vi "Teleop.vi"(10 "Match Info":T1={"Autonomous Elapsed Seconds"=0.0, "TeleOp Elapsed Seconds"=0.0, "Disabled Elapsed Seconds"=0.0, "Visited Autonomous"=FALSE, "Visited TeleOp"=FALSE, "Visited Disabled"=FALSE, "Autonomous Settings"={"Autonomous Style"=enum."Independent", "VI Refnum"=refnum}}, 11 "Call Context":T2) -> ()   [LabVIEW 2017]
doc: "This VI is called for each TeleOp packet received from the DS where the robot is not disabled. It is often used to read from the joysticks and update I/O or to update setpoints for timed control loops. It should complete and return within 20 milliseconds or it may miss DS packets."
uses:
  <vilib>/Rock Robotics/WPI/DriverStation/WPI_DriverStationDerivedRobotMode.ctl
  <vilib>/Rock Robotics/WPI/DriverStation/WPI_DriverStationMatch Info.ctl
  <vilib>/Rock Robotics/WPI/Utilities/WPI_GetSetVariantRefNum.vi
  <vilib>/Rock Robotics/Network Tables/NT Write Boolean Array.vi
  <vilib>/Rock Robotics/Network Tables/NT Write Numeric Array.vi
  <vilib>/Rock Robotics/Network Tables/NT Write Boolean.vi
  <vilib>/Rock Robotics/Network Tables/NT Read Boolean.vi
  <vilib>/Rock Robotics/Network Tables/NT Read Number.vi
panel:
  out "Sample Slider 0":dbl(slide) scale=0.0..5.0
  out "Sample Boolean 1":bool
  out "Sample Boolean 0":bool
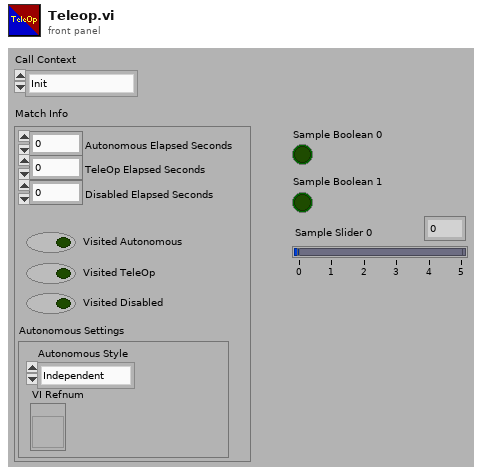
[diagram p1: front panel]
types:
  T1 = typedef "WPI_DriverStationMatch Info.ctl" = cluster{"Autonomous Elapsed Seconds":dbl, "TeleOp Elapsed Seconds":dbl, "Disabled Elapsed Seconds":dbl, "Visited Autonomous":bool, "Visited TeleOp":bool, "Visited Disabled":bool, "Autonomous Settings":cluster{"Autonomous Style":enum16{"Iterative", "Independent"}, "VI Refnum":refnum<vi>}}
  T2 = typedef "WPI_DriverStationDerivedRobotMode.ctl" = enum16{"Init", "Execute", "Stop"}
  T3 = typedef "WPI_RobotDriveDevRef.ctl" = cluster{"DevStatus":errorcluster, "Motors[]":T4[], "Square Inputs":bool, "Max Output":dbl}
  T4 = typedef "WPI_MotorControlDeviceRef.ctl" = cluster{"DeviceStatus":errorcluster, "Type":T5, "PWM":cluster{"PWM Channel":T6, "DeadBand":T7}, "CAN":cluster{"Device Number":u8, "SetOutput VI Ref":variant, "GetOutput VI Ref":variant, "Enable VI Ref":variant, "Disable VI Ref":variant, "Data":variant}, "Invert":bool, "DIO PWM":cluster{"PWM \"Enable\" Channel":T6, "DIOChannel":T8, "PWM Rate":dbl}}
  T5 = typedef "WPI_MotorControlType.ctl" = enum16{"PWM", "CAN", "DIO PWM"}
  T6 = typedef "FPGA_DIOPWMChannel.ctl" = enum8{"PWM 0", "PWM 1", "PWM 2", "PWM 3", "PWM 4", "PWM 5", "PWM 6", "PWM 7", "PWM 8", "PWM 9", "PWM MXP 0", "PWM MXP 1", "PWM MXP 2", "PWM MXP 3", "PWM MXP 4", "PWM MXP 5", "PWM MXP 6", "PWM MXP 7", "PWM MXP 8", "PWM MXP 9", "Invalid"}
  T7 = typedef "WPI_PWMDeadband.ctl" = cluster{"Name":string, "maxPositivePwm":i32, "minPositivePwm":i32, "centerPwm":i32, "maxNegativePwm":i32, "minNegativePwm":i32, "angularRange":u16}
  T8 = typedef "FPGA_DIOChannel.ctl" = enum8{"DIO 0", "DIO 1", "DIO 2", "DIO 3", "DIO 4", "DIO 5", "DIO 6", "DIO 7", "DIO 8", "DIO 9", "DIO MXP 0", "DIO MXP 1", "DIO MXP 2", "DIO MXP 3", "DIO MXP 4", "DIO MXP 5", "DIO MXP 6", "DIO MXP 7", "DIO MXP 8", "DIO MXP 9", "DIO MXP 10", "DIO MXP 11", "DIO MXP 12", "DIO MXP 13", "DIO MXP 14", "DIO MXP 15", "SPI Port CS1", "SPI Port CS2", "SPI Port CS3", "SPI Port MISO", "SPI Port MOSI", "Invalid"}
  T9 = typedef "WPI_JoystickDevRef.ctl" = cluster{"Device":T10}
  T10 = typedef "WPI_JoystickDeviceEnum.ctl" = enum16{"USB 0", "USB 1", "USB 2", "USB 3", "USB 4", "USB 5"}
  T11 = typedef "WPI_SwitchDevRef.ctl" = cluster{"DevStatus":errorcluster, "DIO Channel":T8, "CntIndex":T12, "Normally Closed":bool}
  T12 = typedef "FPGA_CounterCtrSystemIndex.ctl" = enum8{"Ctr 0", "Ctr 1", "Ctr 2", "Ctr 3", "Ctr 4", "Ctr 5", "Ctr 6", "Ctr 7", "Invalid"}
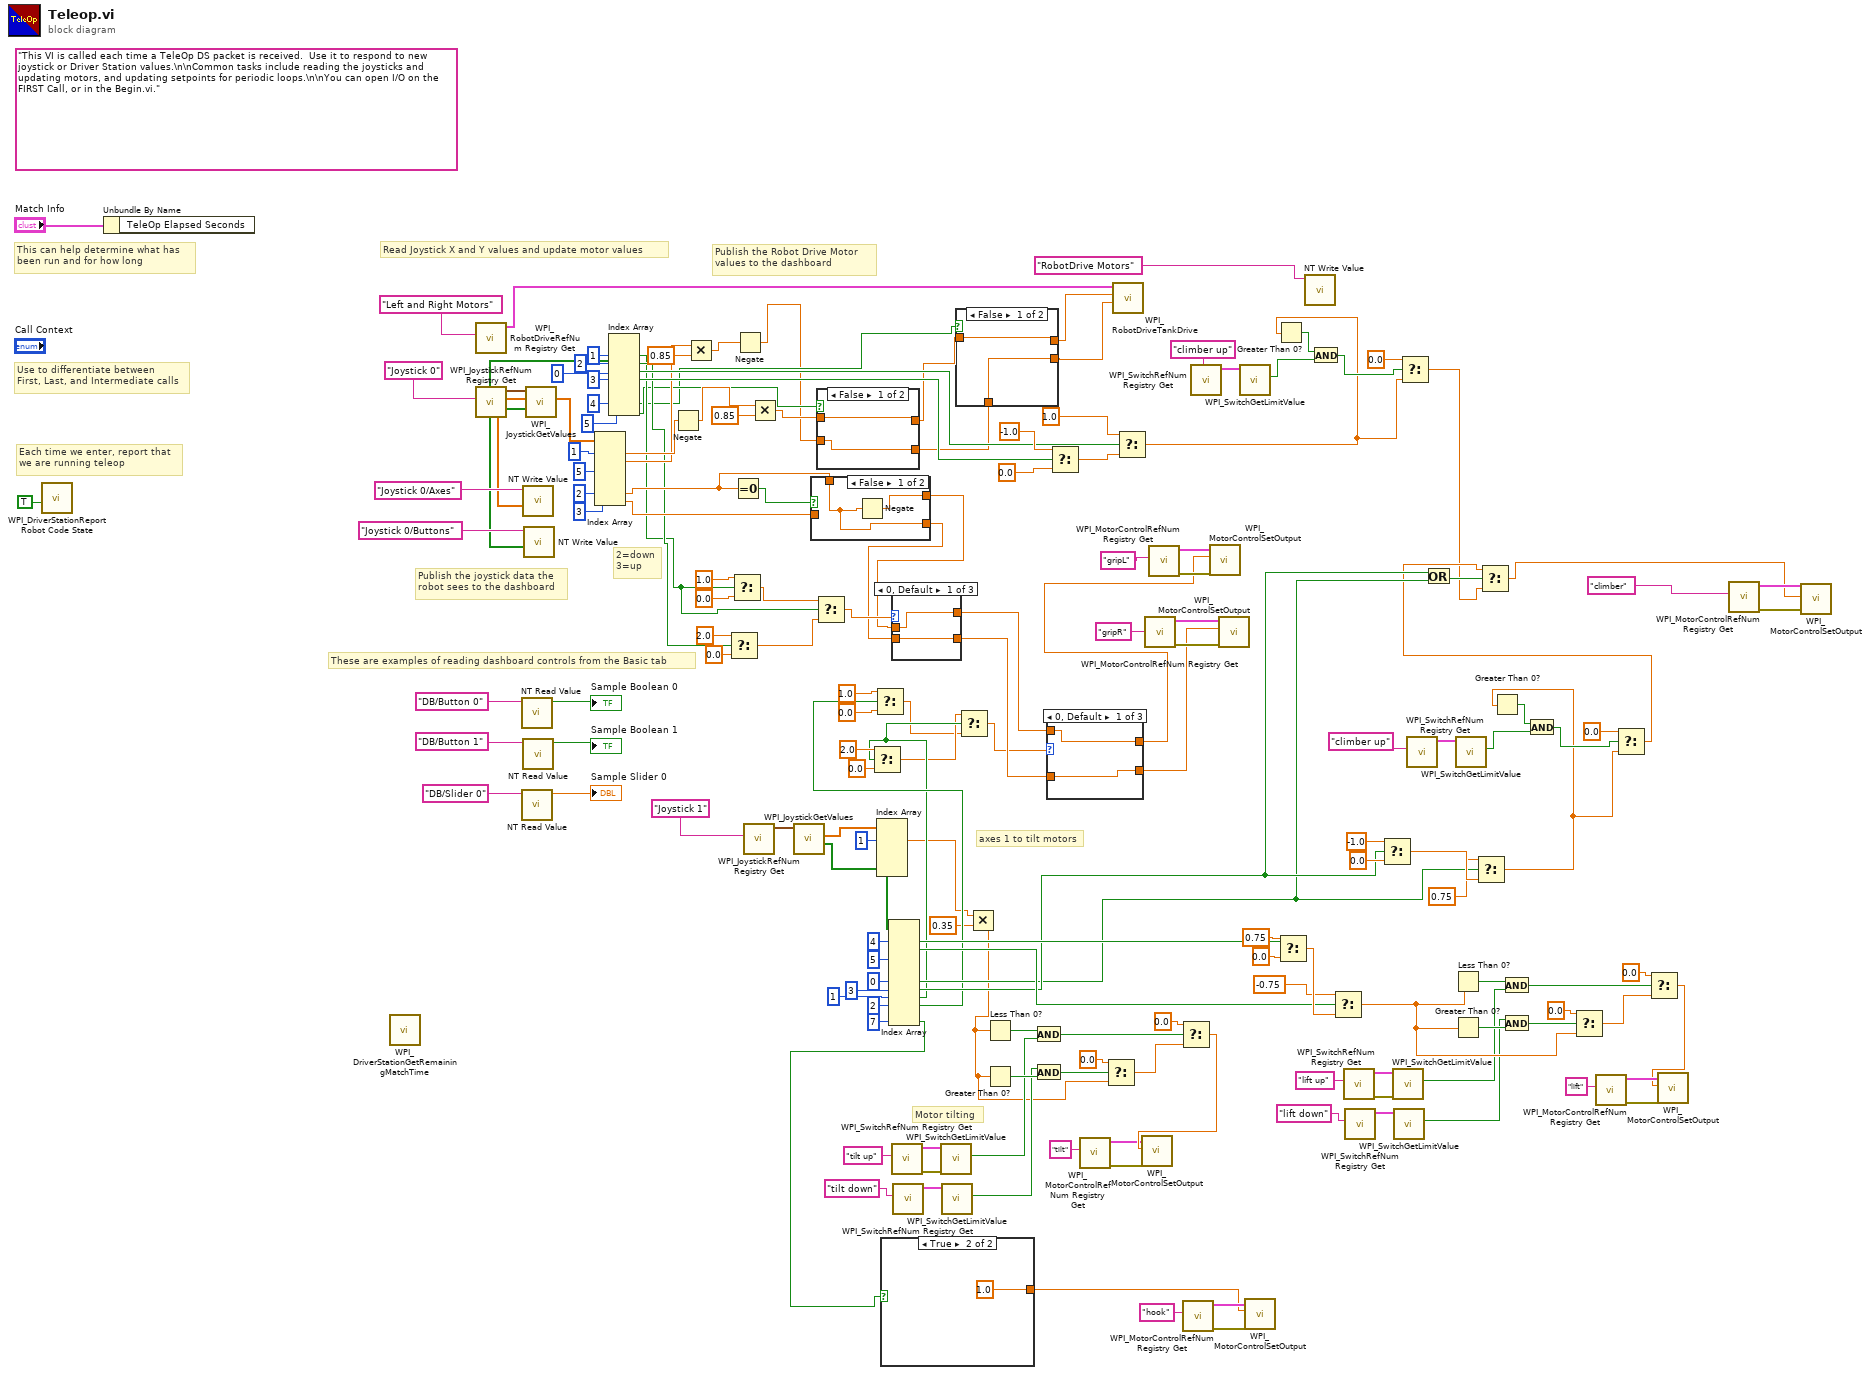
[diagram p0: block diagram]
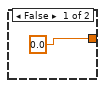
[diagram p2: hidden frame]
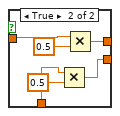
[diagram p3: hidden frame]
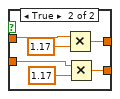
[diagram p4: hidden frame]
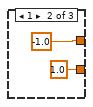
[diagram p5: hidden frame]
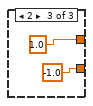
[diagram p6: hidden frame]
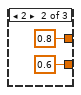
[diagram p7: hidden frame]
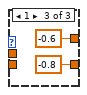
[diagram p8: hidden frame]
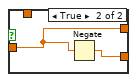
[diagram p9: hidden frame]
diagram:
  (unwired) "This VI is called each time a TeleOp DS packet is received.  Use it to respond to new joystick or Driver Station values.\n\nCommon tasks include reading the joysticks and updating motors, and updating setpoints for periodic loops.\n\nYou can open I/O on the FIRST Call, or in the Begin.vi."
  # "Motor tilting"
  # "axes 1 to tilt motors"
  # "2=down\n3=up"
  # "These are examples of reading dashboard controls from the Basic tab"
  # "Publish the Robot Drive Motor\nvalues to the dashboard"
  # "Publish the joystick data the\nrobot sees to the dashboard"
  # "Each time we enter, report that\nwe are running teleop"
  # "Use to differentiate between\nFirst, Last, and Intermediate calls"
  # "This can help determine what has\nbeen run and for how long"
  # "Read Joystick X and Y values and update motor values"
  n1 = call <vilib>:"WPI_DriverStationReport Robot Code State.vi"("TeleOp"=TRUE ("Autonomous")) -> ()  [unwired: 10 in, 1 out]
  n2 = Unbundle By Name("Match Info") -> ()  [unwired: 1 out]
  n3 = call <vilib>:"WPI_DriverStationGetRemainingMatchTime.vi"() -> ()  [unwired: 10 in, 2 out]
  n4 = call <vilib>:"WPI_RobotDriveRefNum Registry Get.vi"("refnum name"="Left and Right Motors") -> ("RobotDriveDevRef"=w1:T3)  [unwired: 1 in, 9 out]
  n5 = call <vilib>:"WPI_JoystickRefNum Registry Get.vi"("refnum name"="Joystick 0") -> ("JoystickDevRef"=w167:T9)  [unwired: 1 in, 9 out]
  n6 = call-poly <vilib>:"NT Read Value.vi"("Name"="DB/Button 0" ("refnum name")) -> ("Boolean"=→"Sample Boolean 0":bool)  [unwired: 9 in, 1 out]
  n7 = call-poly <vilib>:"NT Read Value.vi"("Name"="DB/Slider 0" ("refnum name")) -> ("Numeric"=→"Sample Slider 0":dbl)  [unwired: 9 in, 1 out]
  n8 = call-poly <vilib>:"NT Read Value.vi"("Name"="DB/Button 1" ("refnum name")) -> ("Boolean"=→"Sample Boolean 1":bool)  [unwired: 9 in, 1 out]
  n9 = call <vilib>:"WPI_JoystickGetValues.vi"("JoystickDevRef"=w167) -> ("Buttons"=w151:bool[], "Axes"=w163:dbl[])  [unwired: 6 in, 3 out]
  n10 = call-poly <vilib>:"NT Write Value.vi"("Numeric Array"=w163, "Name"="Joystick 0/Axes") -> ()  [unwired: 9 in, 1 out]
  n11 = call-poly <vilib>:"NT Write Value.vi"("Boolean Array"=w151, "Name"="Joystick 0/Buttons") -> ()  [unwired: 9 in, 1 out]
  n12 = Index Array(array=w163, index #1=1 ("index"), index #2=5 ("index"), index #6=2 ("index"), index #7=3 ("index")) -> (element #1=w138:dbl, element #2=w129:dbl, element #6=w132:dbl, element #7=w133:dbl)  [unwired: 3 in, 3 out]
  n13 = Index Array(array=w151, index #1=1 ("index"), index #2=2 ("index"), index #3=0 ("index"), index #4=3 ("index"), index #7=4 ("index"), index #8=5 ("index")) -> (element #1=w58:bool, element #2=w61:bool, element #3=w139:bool, element #4=w146:bool, element #7=w44:bool, element #8=w47:bool)  [unwired: 2 in, 2 out]
  n14 = Negate(x=w138) -> (-x=w131:dbl)
  n15 = Multiply(x=w129, y=0.85) -> (x*y=w127:dbl)
  n16 = Select(t=2.0, s=w61, f=0.0) -> (s? t:f=w62:dbl)
  n17 = Select(t=1.0, s=w58, f=0.0) -> (s? t:f=w63:dbl)
  n18 = Equal To 0?(x=w132) -> (x = 0?=w134:bool)
  n19 = Negate(x=w127) -> (-x=w43:dbl)
  n20 = call <vilib>:"WPI_JoystickRefNum Registry Get.vi"("refnum name"="Joystick 1") -> ("JoystickDevRef"=w154:T9)  [unwired: 1 in, 9 out]
  n21 = Multiply(x=w131, y=0.85) -> (x*y=w46:dbl)
  n22 = call <vilib>:"WPI_JoystickGetValues.vi"("JoystickDevRef"=w154) -> ("Buttons"=w97:bool[], "Axes"=w153:dbl[])  [unwired: 6 in, 3 out]
  n23 = case shown="False" w134 {
    tunnel: [w172 w174] -> w56
    tunnel: w133 -> [_ w174]
    tunnel: w132 -> [w171 _]
    tunnel: [w171 w173] -> w55
    frame False {
      n24 = Negate(x=w171) -> (-x=w172:dbl)
    }
    frame True {
      n25 = Negate(x=w174) -> (-x=w173:dbl)
    }
  }
  n26 = Select(t=w63, s=w58, f=w62) -> (s? t:f=w57:dbl)
  n27 = case shown="False" w47 {
    tunnel: w46 -> [w176 w182]
    tunnel: [w176 w180] -> w45
    tunnel: w43 -> [w175 w178]
    tunnel: [w175 w177] -> w2
    frame False {
    }
    frame True {
      n28 = Multiply(x=w182, y=1.17) -> (x*y=w180:dbl)
      n29 = Multiply(x=w178, y=1.17) -> (x*y=w177:dbl)
    }
  }
  n30 = Index Array(array=w153, index #1=1 ("index")) -> (element #1=w7:dbl)  [unwired: 4 in, 4 out]
  n31 = Index Array(array=w97, index #1=4 ("index"), index #2=5 ("index"), index #6=0 ("index"), index #7=3 ("index"), index #8=1 ("index"), index #9=2 ("index"), index #11=7 ("index")) -> (element #1=w94:bool, element #2=w93:bool, element #6=w74:bool, element #7=w75:bool, element #8=w36:bool, element #9=w37:bool, element #11=w9:bool)  [unwired: 4 in, 4 out]
  n32 = Select(t=2.0, s=w36, f=0.0) -> (s? t:f=w15:dbl)
  n33 = Select(t=1.0, s=w37, f=0.0) -> (s? t:f=w14:dbl)
  n34 = case shown="True" w9 {
    tunnel: [0.0 ("Output") 1.0 ("Output")] -> w8
    frame False {
    }
    frame True {
    }
  }
  n35 = case shown="0, Default" w57 {
    tunnel: [w186 0.8 ("upper limit") -0.6 ("upper limit")] -> w52
    tunnel: w56 -> [w186 _ _]
    tunnel: [w185 0.6 ("upper limit") -0.8 ("upper limit")] -> w50
    tunnel: w55 -> [w185 _ _]
    frame 0, Default {
    }
    frame 2 {
    }
    frame 1 {
    }
  }
  n36 = call <vilib>:"WPI_SwitchRefNum Registry Get.vi"("refnum name"="tilt up") -> ("error out"=w33:errorcluster, "SwitchDevRef"=w32:T11)  [unwired: 9 in]
  n37 = call <vilib>:"WPI_SwitchRefNum Registry Get.vi"("refnum name"="tilt down") -> ("SwitchDevRef"=w31:T11)  [unwired: 9 in, 1 out]
  n38 = call <vilib>:"WPI_SwitchGetLimitValue.vi"("error in (no error)"=w33, "SwitchDevRef"=w32) -> ("Switch Pressed"=w18:bool)  [unwired: 7 in, 2 out]
  n39 = call <vilib>:"WPI_SwitchGetLimitValue.vi"("SwitchDevRef"=w31) -> ("Switch Pressed"=w19:bool)  [unwired: 8 in, 2 out]
  n40 = case shown="False" w44 {
    tunnel: w45 -> [w192 w198]
    tunnel: [w192 w196] -> w4
    tunnel: [w191 w193] -> w3
    tunnel: w2 -> [w191 w194]
    frame False {
    }
    frame True {
      n41 = Multiply(x=w194, y=0.5) -> (x*y=w193:dbl)
      n42 = Multiply(x=w198, y=0.5) -> (x*y=w196:dbl)
    }
  }
  n43 = Select(t=w15, s=w36, f=w14) -> (s? t:f=w35:dbl)
  n44 = Multiply(x=w7, y=0.35) -> (x*y=w6:dbl)
  n45 = Less Than 0?(x=w6) -> (x < 0?=w23:bool)
  n46 = Greater Than 0?(x=w6) -> (x > 0?=w24:bool)
  n47 = And(x=w23, y=w18) -> (x .and. y?=w25:bool)
  n48 = And(x=w19, y=w24) -> (x .and. y?=w26:bool)
  n49 = case shown="0, Default" w35 {
    tunnel: [w199 -1.0 ("upper limit") 1.0 ("upper limit")] -> w53
    tunnel: w52 -> [w199 _ _]
    tunnel: [w200 1.0 ("upper limit") -1.0 ("upper limit")] -> w51
    tunnel: w50 -> [w200 _ _]
    frame 0, Default {
    }
    frame 1 {
    }
    frame 2 {
    }
  }
  n50 = Select(t=-1.0, s=w146, f=0.0) -> (s? t:f=w143:dbl)
  n51 = call <vilib>:"WPI_MotorControlRefNum Registry Get.vi"("refnum name"="tilt") -> ("error out"=w27:errorcluster, "MotorControlDevRef"=w16:T4)  [unwired: 9 in]
  n52 = Select(t=0.0, s=w26, f=w6) -> (s? t:f=w20:dbl)
  n53 = call <vilib>:"WPI_RobotDriveTankDrive.vi"("Right axis value"=w3, "Left axis value"=w4, "RobotDriveDevRef"=w1) -> ()  [unwired: 6 in, 3 out]
  n54 = Select(t=1.0, s=w139, f=w143) -> (s? t:f=w120:dbl)
  n55 = call <vilib>:"WPI_MotorControlRefNum Registry Get.vi"("refnum name"="gripR") -> ("error out"=w69:errorcluster, "MotorControlDevRef"=w49:T4)  [unwired: 9 in]
  n56 = call <vilib>:"WPI_MotorControlRefNum Registry Get.vi"("refnum name"="gripL") -> ("error out"=w135:errorcluster, "MotorControlDevRef"=w136:T4)  [unwired: 9 in]
  n57 = Select(t=0.0, s=w25, f=w20) -> (s? t:f=w17:dbl)
  n58 = call <vilib>:"WPI_MotorControlSetOutput.vi"("error in (no error)"=w27, "Output"=w17, "MotorControlDevRef"=w16) -> ()  [unwired: 6 in, 3 out]
  n59 = call <vilib>:"WPI_MotorControlRefNum Registry Get.vi"("refnum name"="hook") -> ("error out"=w12:errorcluster, "MotorControlDevRef"=w11:T4)  [unwired: 9 in]
  n60 = call <vilib>:"WPI_SwitchRefNum Registry Get.vi"("refnum name"="climber up") -> ("SwitchDevRef"=w126:T11)  [unwired: 9 in, 1 out]
  n61 = call <vilib>:"WPI_MotorControlSetOutput.vi"("error in (no error)"=w135, "Output"=w53, "MotorControlDevRef"=w136) -> ()  [unwired: 6 in, 3 out]
  n62 = call <vilib>:"WPI_MotorControlSetOutput.vi"("error in (no error)"=w69, "Output"=w51, "MotorControlDevRef"=w49) -> ()  [unwired: 6 in, 3 out]
  n63 = call <vilib>:"WPI_SwitchGetLimitValue.vi"("SwitchDevRef"=w126) -> ("Switch Pressed"=w124:bool)  [unwired: 8 in, 2 out]
  n64 = call <vilib>:"WPI_MotorControlSetOutput.vi"("error in (no error)"=w12, "Output"=w8, "MotorControlDevRef"=w11) -> ()  [unwired: 6 in, 3 out]
  n65 = Greater Than 0?(x=w120) -> (x > 0?=w123:bool)
  n66 = Select(t=0.75, s=w94, f=0.0) -> (s? t:f=w114:dbl)
  n67 = call-poly <vilib>:"NT Write Value.vi"("Name"="RobotDrive Motors") -> ()  [unwired: 10 in, 1 out]
  n68 = And(x=w123, y=w124) -> (x .and. y?=w121:bool)
  n69 = Select(t=-0.75, s=w93, f=w114) -> (s? t:f=w105:dbl)
  n70 = call <vilib>:"WPI_SwitchRefNum Registry Get.vi"("refnum name"="lift up") -> ("error out"=w103:errorcluster, "SwitchDevRef"=w102:T11)  [unwired: 9 in]
  n71 = call <vilib>:"WPI_SwitchRefNum Registry Get.vi"("refnum name"="lift down") -> ("SwitchDevRef"=w101:T11)  [unwired: 9 in, 1 out]
  n72 = Select(t=-1.0, s=w75, f=0.0) -> (s? t:f=w87:dbl)
  n73 = call <vilib>:"WPI_SwitchGetLimitValue.vi"("error in (no error)"=w103, "SwitchDevRef"=w102) -> ("Switch Pressed"=w99:bool)  [unwired: 7 in, 2 out]
  n74 = call <vilib>:"WPI_SwitchGetLimitValue.vi"("SwitchDevRef"=w101) -> ("Switch Pressed"=w98:bool)  [unwired: 8 in, 2 out]
  n75 = Select(t=0.0, s=w121, f=w120) -> (s? t:f=w71:dbl)
  n76 = call <vilib>:"WPI_SwitchRefNum Registry Get.vi"("refnum name"="climber up") -> ("SwitchDevRef"=w85:T11)  [unwired: 9 in, 1 out]
  n77 = Or(x=w75, y=w74) -> (x .or. y?=w73:bool)
  n78 = Less Than 0?(x=w105) -> (x < 0?=w109:bool)
  n79 = Greater Than 0?(x=w105) -> (x > 0?=w110:bool)
  n80 = call <vilib>:"WPI_SwitchGetLimitValue.vi"("SwitchDevRef"=w85) -> ("Switch Pressed"=w83:bool)  [unwired: 8 in, 2 out]
  n81 = Select(t=0.75, s=w74, f=w87) -> (s? t:f=w79:dbl)
  n82 = Greater Than 0?(x=w79) -> (x > 0?=w82:bool)
  n83 = And(x=w109, y=w99) -> (x .and. y?=w111:bool)
  n84 = And(x=w98, y=w110) -> (x .and. y?=w112:bool)
  n85 = And(x=w82, y=w83) -> (x .and. y?=w80:bool)
  n86 = Select(t=0.0, s=w112, f=w105) -> (s? t:f=w106:dbl)
  n87 = call <vilib>:"WPI_MotorControlRefNum Registry Get.vi"("refnum name"="lift") -> ("error out"=w117:errorcluster, "MotorControlDevRef"=w118:T4)  [unwired: 9 in]
  n88 = Select(t=0.0, s=w80, f=w79) -> (s? t:f=w72:dbl)
  n89 = Select(t=w72, s=w73, f=w71) -> (s? t:f=w70:dbl)
  n90 = Select(t=0.0, s=w111, f=w106) -> (s? t:f=w104:dbl)
  n91 = call <vilib>:"WPI_MotorControlSetOutput.vi"("error in (no error)"=w117, "Output"=w104, "MotorControlDevRef"=w118) -> ()  [unwired: 6 in, 3 out]
  n92 = call <vilib>:"WPI_MotorControlRefNum Registry Get.vi"("refnum name"="climber") -> ("error out"=w90:errorcluster, "MotorControlDevRef"=w91:T4)  [unwired: 9 in]
  n93 = call <vilib>:"WPI_MotorControlSetOutput.vi"("error in (no error)"=w90, "Output"=w70, "MotorControlDevRef"=w91) -> ()  [unwired: 6 in, 3 out]
